vi "Show Unable to Start Stream Error Dialog.vi"(8 "error in (no error)":errorcluster, 9 "Stream Start Error":errorcluster, 11 "UI in":refnum<class "UI.lvclass">) -> (0 "error out":errorcluster)   [LabVIEW 2020, in "AR Example.lvlib" / "UI.lvclass"]
uses:
  UI.lvclass
  <vilib>/Utility/error.llb/DialogType.ctl
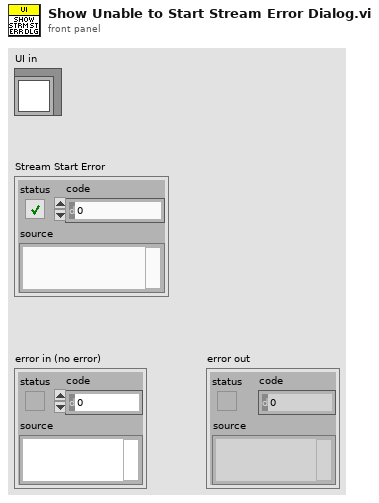
[diagram p1: front panel]
types:
  T1 = typedef "DialogType.ctl" = u16
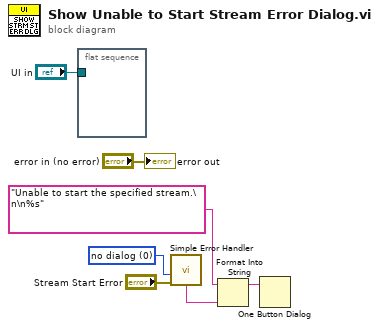
[diagram p0: block diagram]
diagram:
  w3 = T1 0 items=["no dialog", "OK message", "continue or stop message", "OK message + warnings", "continue/stop + warnings"] ("type of dialog (OK msg:1)")
  n1 = flat-sequence {
    tunnel: "UI in" -> [_]
    frame #0 {
    }
  }
  n2 = call <vilib>:"Simple Error Handler.vi"("type of dialog (OK msg:1)"=w3, "error in (no error)"="Stream Start Error") -> ("message"=w1:string)  [unwired: 3 in, 4 out]
  n3 = Format Into String(initial string="Unable to start the specified stream.\n\n%s" ("message"), w1) -> (resulting string=w2:string)  [unwired: 2 in, 1 out]
  n4 = One Button Dialog(message=w2) -> ()  [unwired: 1 in, 1 out]
  "error out" <- "error in (no error)"
